vi "motorGroupSettings.vi"(8 "error in (no error)":errorcluster, 9 "Velocity (units/s) in":dbl min=0.0 format="%.4g", 10 "Acceleration (0 units/s²) in":dbl min=0.0 format="%.4g", 11 "VISA Refnum in":refnum<visa-resource-name>) -> (0 "error out":errorcluster, 3 "VISA Refnum out":refnum<visa-resource-name>)   [LabVIEW 2014]
doc: "Newport Motion Controler\n\nSettings Velocity and Acceleration at Group\n\nAndré Romero - 2020\nandretec@ifsc.usp.br"
uses:
  <userlib>/Newport ESP301/Newport ESP301.lvlib
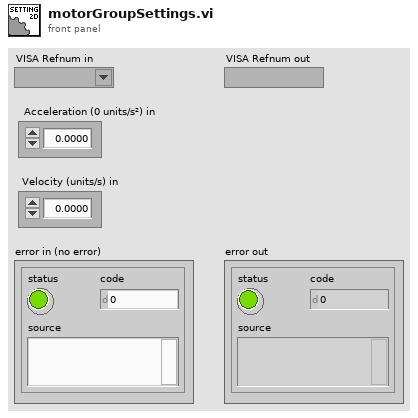
[diagram p1: front panel]
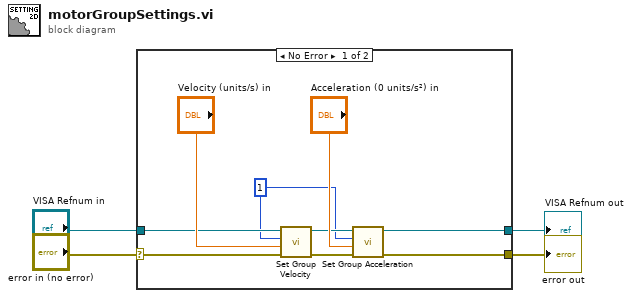
[diagram p0: block diagram]
diagram:
  n1 = case shown="No Error" "error in (no error)" {
    selector: "error in (no error)" -> [w5 w14]
    tunnel: [w10 w14] -> w4
    tunnel: [w9 w15] -> w3
    tunnel: "VISA Refnum in" -> [w7 w15]
    frame No Error {
      w6 = 1 ("Group #")
      n2 = call <userlib>:"Set Group Velocity.vi"("error in (no error)"=w5, "Velocity (units/s)"="Velocity (units/s) in", "Group Number (1)"=w6, "VISA resource name"=w7) -> ("error out"=w11:errorcluster, "VISA resource name out"=w8:refnum<visa-resource-name>)  [unwired: 2 in]
      n3 = call <userlib>:"Set Group Acceleration.vi"("error in (no error)"=w11, "Acceleration (0 units/s²)"="Acceleration (0 units/s²) in", "Group Number (1)"=w6, "VISA resource name"=w8) -> ("error out"=w10:errorcluster, "VISA resource name out"=w9:refnum<visa-resource-name>)  [unwired: 2 in]
    }
    frame Error {
    }
  }
  "error out" <- w4
  "VISA Refnum out" <- w3
